vi "Main.vi"() -> ()   [LabVIEW 2014]
uses:
  Controls/Address.ctl
  Controls/States.ctl
  Controls/Property.ctl
  Controls/FP Control Refs.ctl
  Controls/Data.ctl
  Controls/Operator.ctl
  Controls/Filter Criteria.ctl
  Controls/Fields.ctl
  SubVIs/Web/Search String Type.ctl
  Controls/Sort Order.ctl
  Controls/Config Settings.ctl
  Controls/Web Filter Cluster.ctl
panel:
  out "Status":string
  in  "Data":T1
  in  "Hide Button":bool
  in  "Filter Button":bool
  in  "Delete Button":bool
  out "Results Listbox":i32(listbox)
  in  "Search Button":bool
  in  "Save As Button":bool
  in  "Search Box":string
  out "error out":errorcluster
  in  "error in":errorcluster
  in  "States":T12=enum."Convert to Searchable Web Address"
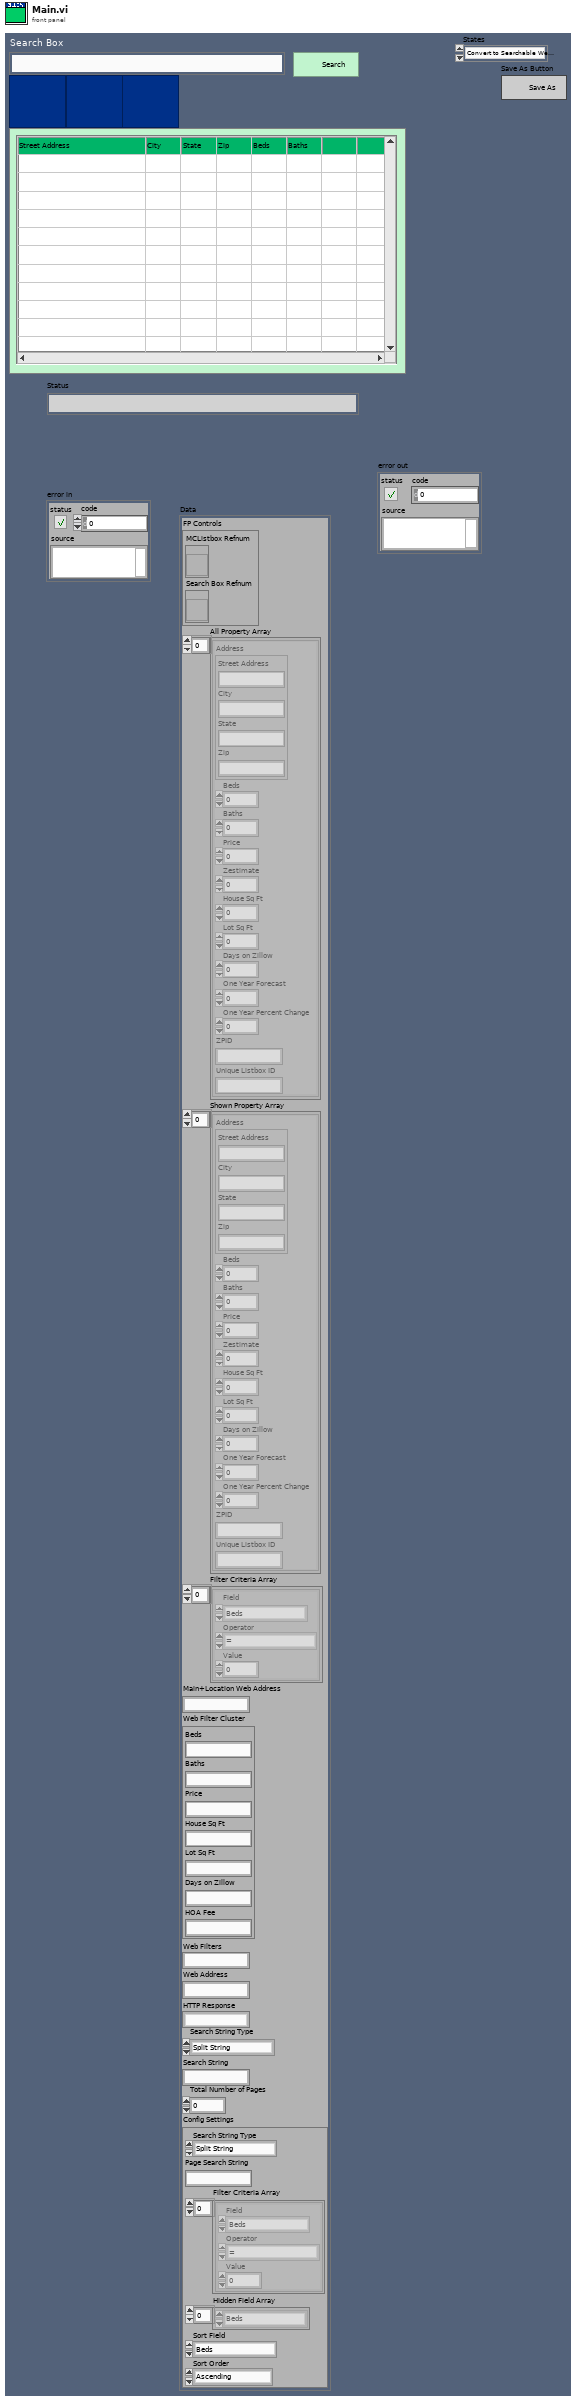
[diagram p1: front panel]
types:
  T1 = typedef "Data.ctl" = cluster{"FP Controls":T2, "All Property Array":T3[], "Shown Property Array":T3[], "Filter Criteria Array":T5[], "Main+Location Web Address":string, "Web Filter Cluster":T8, "Web Filters":string, "Web Address":string, "HTTP Response":string, "Search String Type":T9, "Search String":string, "Total Number of Pages":i32, "Config Settings":T10}
  T2 = typedef "FP Control Refs.ctl" = cluster{"MCListbox Refnum":refnum<vi>, "Search Box Refnum":refnum<vi>}
  T3 = typedef "Property.ctl" = cluster{"Address":T4, "Beds":dbl, "Baths":dbl, "Price":dbl, "Zestimate":dbl, "House Sq Ft":dbl, "Lot Sq Ft":dbl, "Days on Zillow":dbl, "One Year Forecast":dbl, "One Year Percent Change":dbl, "ZPID":string, "Unique Listbox ID":string}
  T4 = typedef "Address.ctl" = cluster{"Street Address":string, "City":string, "State":string, "Zip":string}
  T5 = typedef "Filter Criteria.ctl" = cluster{"Field":T6, "Operator":T7, "Value":dbl}
  T6 = typedef "Fields.ctl" = enum16{"Beds", "Baths", "Price", "Zestimate", "House Sq Ft", "Lot Sq Ft", "Days on Zillow", "One Year Forecast", "One Year Percent Change", "Deal Ratio"}
  T7 = typedef "Operator.ctl" = enum16{"=", ">=", "<=", "!="}
  T8 = typedef "Web Filter Cluster.ctl" = cluster{"Beds":string, "Baths":string, "Price":string, "House Sq Ft":string, "Lot Sq Ft":string, "Days on Zillow":string, "HOA Fee":string}
  T9 = typedef "Search String Type.ctl" = enum16{"Split String", "Match Pattern", "Match RegEx"}
  T10 = typedef "Config Settings.ctl" = cluster{"Search String Type":T9, "Page Search String":string, "Filter Criteria Array":T5[], "Hidden Field Array":T6[], "Sort Field":T6, "Sort Order":T11}
  T11 = typedef "Sort Order.ctl" = enum16{"Ascending", "Descending"}
  T12 = typedef "States.ctl" = enum16{"Read Config File", "Convert to Searchable Web Address", "Submit HTTP Request", "Get Total Pages", "Parse Info from Main Page", "Check if Last Page", "Iterate Page", "Check if Property Exists in DB", "Exit"}
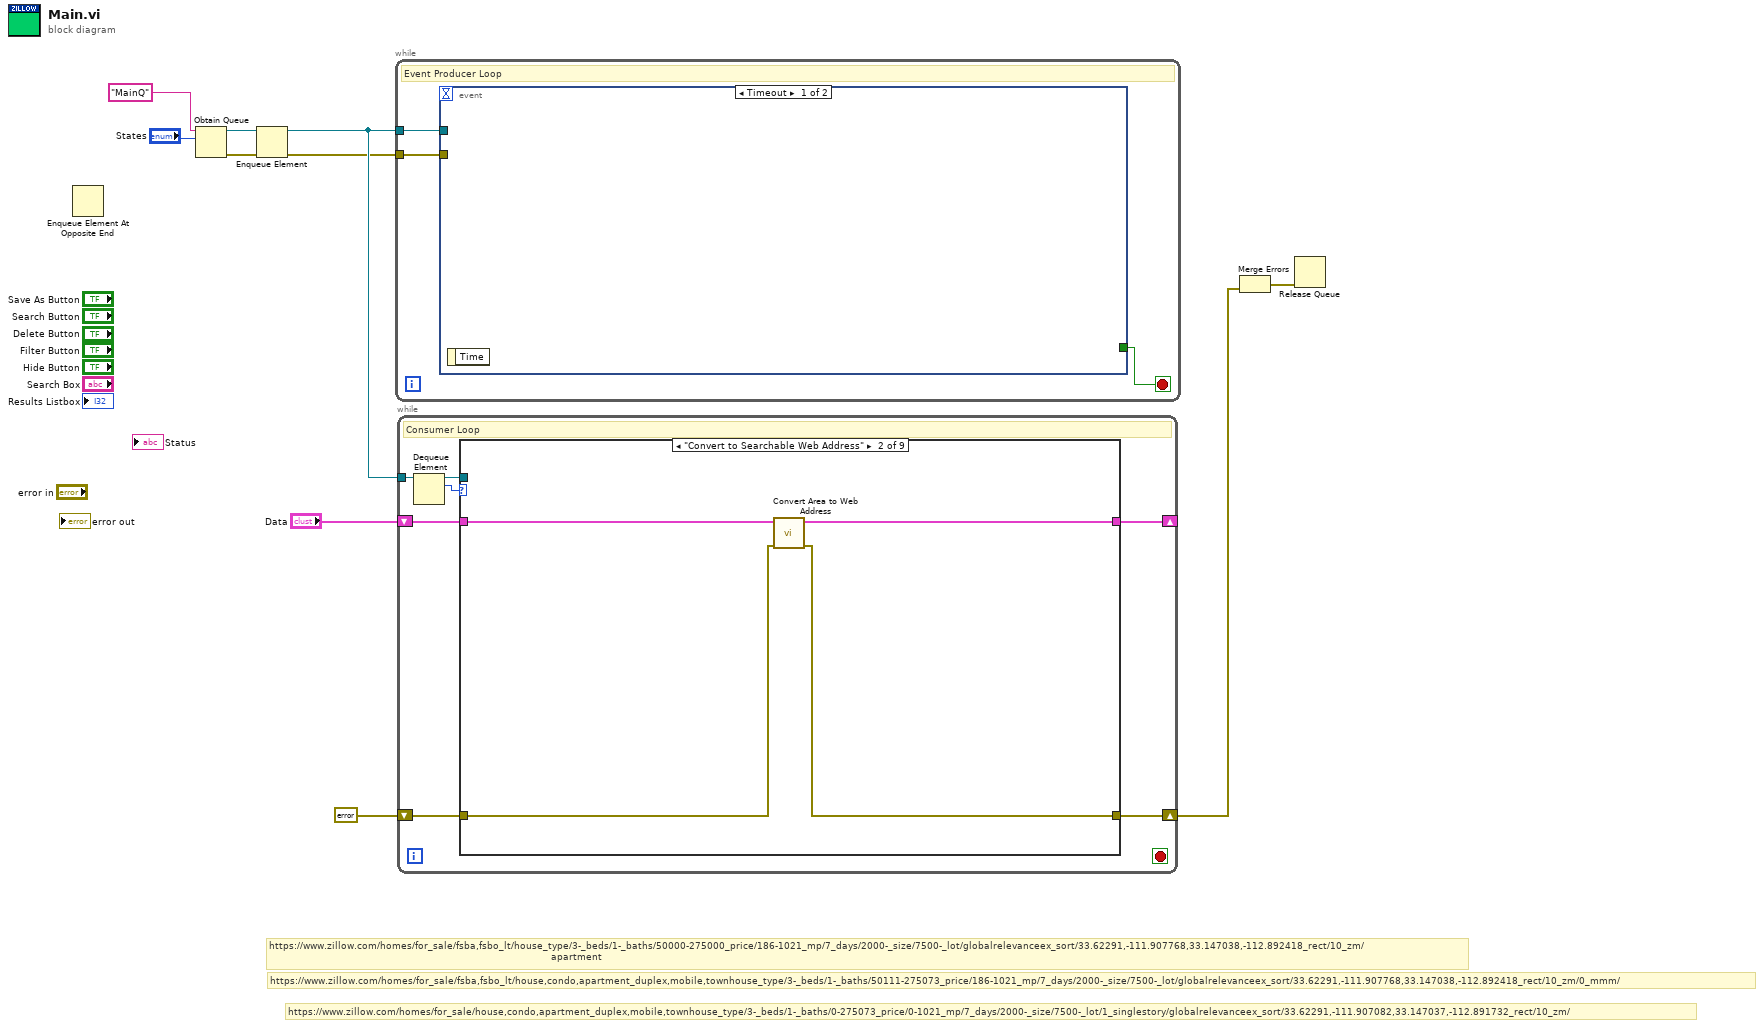
[diagram p0: block diagram]
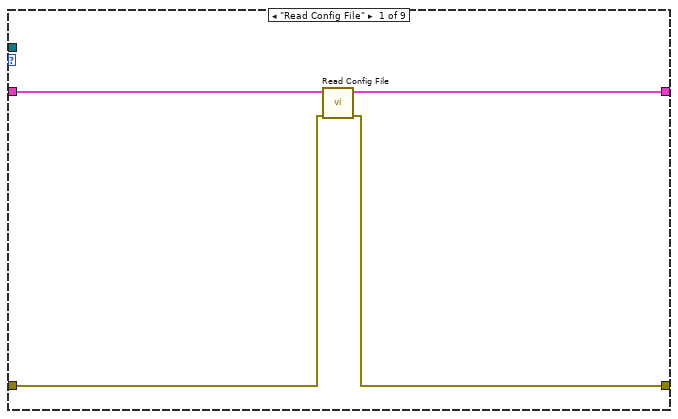
[diagram p2: hidden frame]
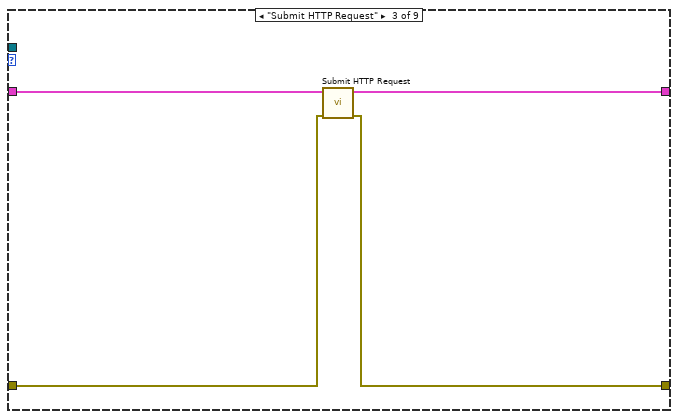
[diagram p3: hidden frame]
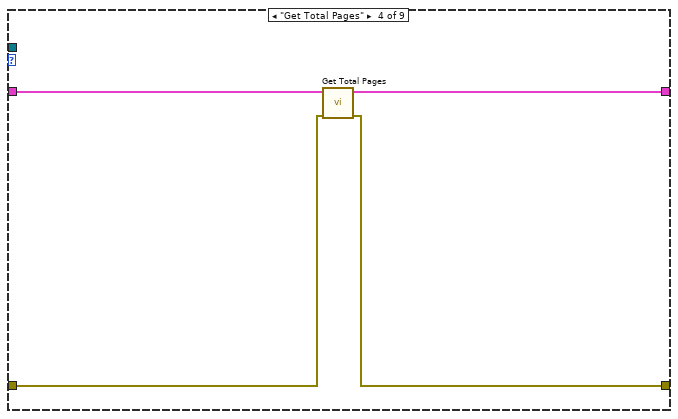
[diagram p4: hidden frame]
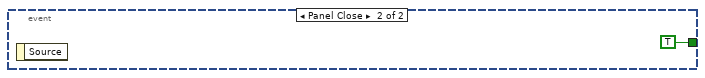
[diagram p10: hidden frame]
diagram:
  # "https://www.zillow.com/homes/for_sale/house,condo,apartment_duplex,mobile,townhouse_type/3-_beds/1-_baths/0-275073_price/0-1021_mp/7_days/2000-_size/7500-_lot/1_singlestory/globalrelevanceex_sort/33.62291,-111.907082,33.147037,-112.891732_rect/10_zm/"
  # "https://www.zillow.com/homes/for_sale/fsba,fsbo_lt/house,condo,apartment_duplex,mobile,townhouse_type/3-_beds/1-_baths/50111-275073_price/186-1021_mp/7_days/2000-_size/7500-_lot/globalrelevanceex_sort/33.62291,-111.907768,33.147038,-112.892418_rect/10_zm/0_mmm/"
  # "https://www.zillow.com/homes/for_sale/fsba,fsbo_lt/house_type/3-_beds/1-_baths/50000-275000_price/186-1021_mp/7_days/2000-_size/7500-_lot/globalrelevanceex_sort/33.62291,-111.907768,33.147038,-112.892418_rect/10_zm/\n                                                                                              apartment"
  n1 = Enqueue Element At Opposite End() -> ()  [unwired: 4 in, 3 out]
  n2 = Obtain Queue(name (unnamed)="MainQ", element data type="States") -> (queue out=w9:refnum<queue>, error out=w10:errorcluster)  [unwired: 3 in, 1 out]
  n3 = Enqueue Element(queue=w9, error in (no error)=w10) -> (queue out=w8:refnum<queue>, error out=w7:errorcluster)  [unwired: 2 in, 1 out]
  n4 = while {
    tunnel: w8 -> [w13]
    tunnel: w7 -> [w11]
    stop <- w12 stop-if-true
    # "Event Producer Loop"
    n5 = event shown="[0] Timeout" {
      selector: _ -> [_ _]
      dyn-events: _ -> [_ _]
      timeout: _ -> [_ _]
      tunnel: w13 -> [_ _]
      tunnel: [_ TRUE] -> w12
      tunnel: w11 -> [_ _]
      event Timeout {
        n6 = event-data() -> ()  [unwired: 1 in, 1 out]
      }
      event Panel Close {
        n7 = event-data() -> ()  [unwired: 1 in, 1 out]
      }
    }
  }
  n8 = while {
    tunnel: w8 -> [w21]
    shift-right: [w19] -> w5
    shift-left: errorcluster {"status"=FALSE, "code"=0, "source"=""} ("error in") -> [w20]
    shift-right: [w15] -> _
    shift-left: "Data" -> [w16]
    stop <- _ stop-if-true
    # "Consumer Loop"
    n9 = Dequeue Element(queue=w21) -> (queue out=w18:refnum<queue>, element=w17:T12)  [unwired: 2 in, 2 out]
    n10 = case shown="\"Convert to Searchable Web Address\"" w17 {
      tunnel: w20 -> [w23 w27 w31 w35 w38 w40 w42 w44 w46]
      tunnel: [w22 w26 w30 w34 w38 w40 w42 w44 w46] -> w19
      tunnel: w18 -> [_ _ _ _ _ _ _ _ _]
      tunnel: w16 -> [w25 w29 w33 w37 w39 w41 w43 w45 w47]
      tunnel: [w24 w28 w32 w36 w39 w41 w43 w45 w47] -> w15
      frame "Read Config File" {
        n11 = call "Read Config File.vi"("error in"=w23, "Data"=w25) -> ("error out"=w22:errorcluster, "Data Out"=w24:T1)  [unwired: 8 in]
      }
      frame "Convert to Searchable Web Address" {
        n12 = call "Convert Area to Web Address.vi"("error in"=w27, "Data"=w29) -> ("error out"=w26:errorcluster, "Data Out"=w28:T1)  [unwired: 8 in]
      }
      frame "Submit HTTP Request" {
        n13 = call "Submit HTTP Request.vi"("error in"=w31, "Data"=w33) -> ("error out"=w30:errorcluster, "Data Out"=w32:T1)  [unwired: 8 in]
      }
      frame "Get Total Pages" {
        n14 = call "Get Total Pages.vi"("error in"=w35, "Data"=w37) -> ("error out"=w34:errorcluster, "Data Out"=w36:T1)  [unwired: 8 in]
      }
      frame "Parse Info from Main Page" {
      }
      frame "Check if Last Page" {
      }
      frame "Iterate Page" {
      }
      frame "Check if Property Exists in DB" {
      }
      frame "Exit" {
      }
    }
  }
  n15 = Merge Errors(w5) -> (w4:errorcluster)  [unwired: 1 in]
  n16 = Release Queue(error in (no error)=w4) -> ()  [unwired: 2 in, 3 out]
